vi "BRig_dataTrial_L_Wro_event_I_l2.vi"() -> (2 "output_L_Wro_event_I_l2":i32)   [LabVIEW 2014]
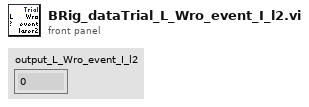
[diagram p1: front panel]
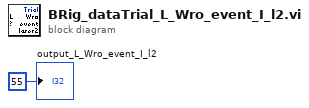
[diagram p0: block diagram]
diagram:
  "output_L_Wro_event_I_l2" <- 55 ("output_iBlock")
